vi "grSim_Replacement.vi"(5 "grSim_RobotReplacement":T1[](array[typedef]), 10 "repalceBall":bool, 11 "grSim_BallReplacement":T2) -> (1 "Array":u8[](array[numeric]))   [LabVIEW 2020]
uses:
  grSim_BallReplacement.ctl
  grSim RobotReplacement.ctl
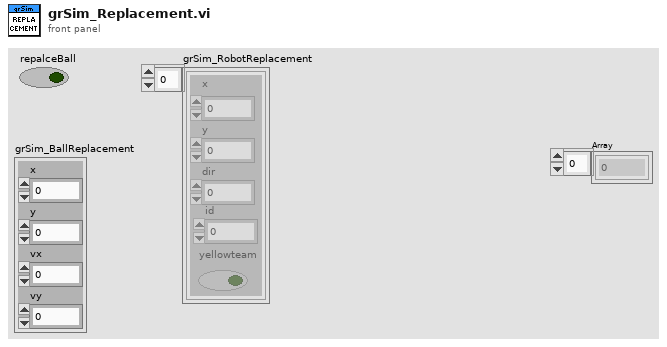
[diagram p1: front panel]
types:
  T1 = typedef "grSim RobotReplacement.ctl" = cluster{"x":dbl, "y":dbl, "dir":dbl, "yellowteam":bool, "id":u32}
  T2 = typedef "grSim_BallReplacement.ctl" = cluster{"x":dbl, "y":dbl, "vx":dbl, "vy":dbl}
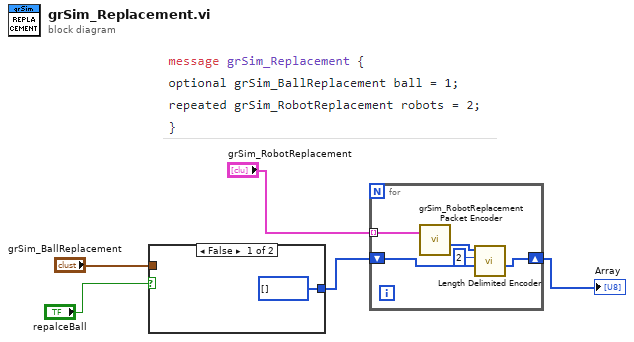
[diagram p0: block diagram]
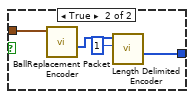
[diagram p2: hidden frame]
diagram:
  n1 = case shown="False" "repalceBall" {
    tunnel: "grSim_BallReplacement" -> [_ w10]
    tunnel: [u8[] [] ("Array") w7] -> w3
    frame False {
    }
    frame True {
      n2 = call "BallReplacement Packet Encoder.vi"("grSim_BallReplacement"=w10) -> ("Array"=w9:u8[])  [unwired: 10 in]
      n3 = call "Length Delimited Encoder.vi"("Key"=u32 1, "Array In 2"=w9) -> ("Array"=w7:u8[])  [unwired: 9 in]
    }
  }
  n4 = for {
    tunnel: "grSim_RobotReplacement" -> [w15] mode=indexing
    shift-right: [w13] -> w2
    shift-left: w3 -> [w14]
    n5 = call "grSim_RobotReplacement Packet Encoder.vi"("grSim_RobotReplacement"=w15) -> ("Array"=w12:u8[])  [unwired: 10 in]
    n6 = call "Length Delimited Encoder.vi"("Array In"=w14, "Key"=u32 2, "Array In 2"=w12) -> ("Array"=w13:u8[])  [unwired: 8 in]
  }
  "Array" <- w2
